vi "data_collector.vi"() -> ()   [LabVIEW 2024]
panel:
  out "Signal":dbl[](graph)
  in  "stop":bool
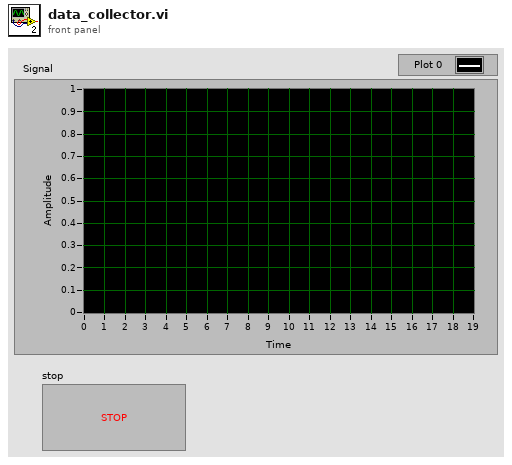
[diagram p1: front panel]
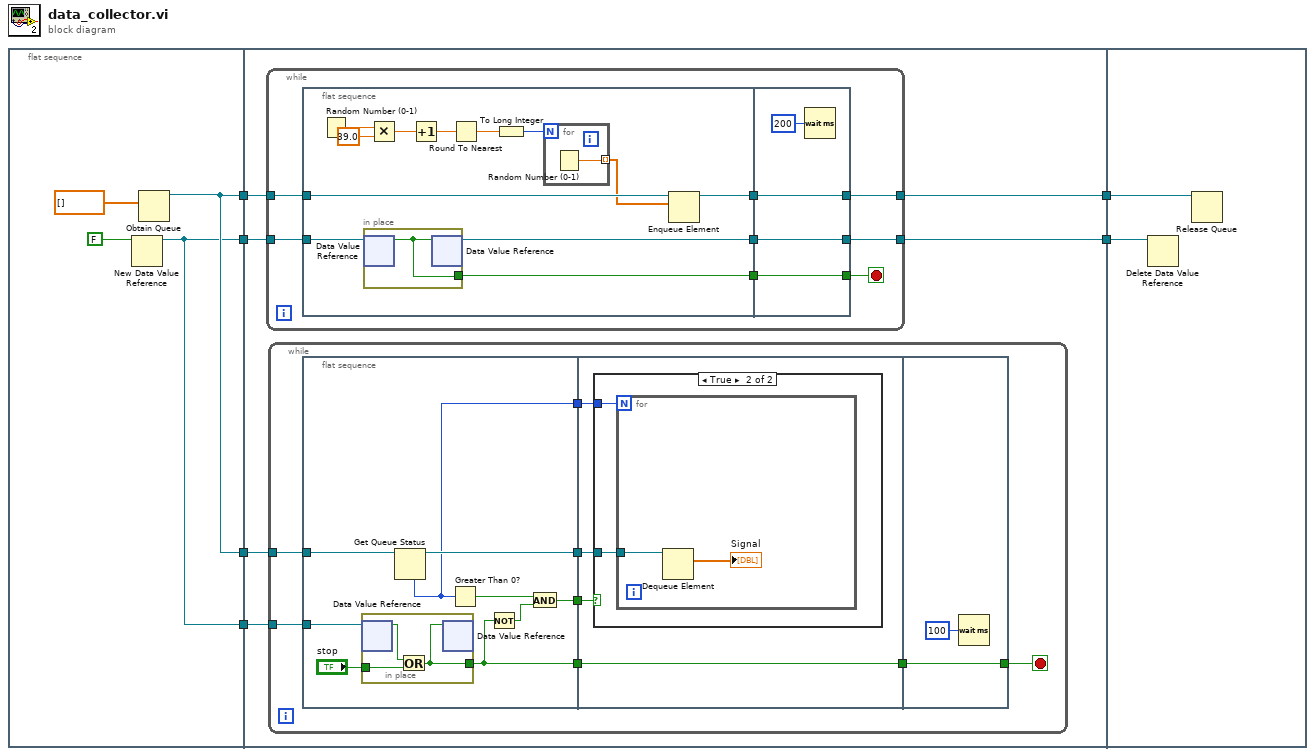
[diagram p0: block diagram]
diagram:
  n1 = flat-sequence {
    tunnel: [w8] -> w6
    tunnel: [w7] -> w5
    tunnel: [w8] -> w3
    tunnel: [w7] -> w2
    tunnel: w6 -> [w16]
    tunnel: w5 -> [w15]
    tunnel: [w14] -> w4
    tunnel: w3 -> [w13]
    tunnel: w2 -> [w12]
    tunnel: [w11] -> w1
    tunnel: w4 -> [w74]
    tunnel: w1 -> [w73]
    frame #0 {
      n2 = New Data Value Reference(data value=FALSE) -> (data value reference=w7:refnum<data-value>)  [unwired: 1 in, 1 out]
      n3 = Obtain Queue(element data type=dbl[] []) -> (queue out=w8:refnum<queue>)  [unwired: 4 in, 2 out]
    }
    frame #1 {
      n4 = while {
        tunnel: w16 -> [w53]
        tunnel: w15 -> [w54]
        tunnel: [w49] -> w14
        tunnel: [w47] -> w11
        stop <- w51 stop-if-true
        n5 = flat-sequence {
          tunnel: w54 -> [w58]
          tunnel: w53 -> [w60]
          tunnel: [w57] -> w52
          tunnel: [w56] -> w50
          tunnel: [w55] -> w48
          tunnel: [w71] -> w51
          tunnel: w52 -> [w71]
          tunnel: [w70] -> w49
          tunnel: w50 -> [w70]
          tunnel: w48 -> [w69]
          tunnel: [w69] -> w47
          frame #0 {
            n6 = Random Number (0-1)() -> (number: 0 to 1=w66:dbl)
            n7 = in-place {
              in-place-border: [w67] -> w57
              n8 = in-place-dvr #1(w58) -> (w67:bool)  [unwired: 1 out]
              n9 = in-place-dvr #1(w67) -> (w55:refnum<data-value>)  [unwired: 1 out]
            }
            n10 = Multiply(x=w66, y=39.0) -> (x*y=w64:dbl)
            n11 = Increment(x=w64) -> (x+1=w63:dbl)
            n12 = Round To Nearest(number=w63) -> (nearest integer value=w62:dbl)
            n13 = To Long Integer(number=w62) -> (32bit integer=w61:i32)
            n14 = for {
              N: w61 -> [_]
              tunnel: [w68] -> w59 mode=indexing
              n15 = Random Number (0-1)() -> (number: 0 to 1=w68:dbl)
            }
            n16 = Enqueue Element(queue=w60, element=w59) -> (queue out=w56:refnum<queue>)  [unwired: 2 in, 2 out]
          }
          frame #1 {
            n17 = Wait (ms)(milliseconds to wait=u32 200) -> ()  [unwired: 1 out]
          }
        }
      }
      n18 = while {
        tunnel: w13 -> [w24]
        tunnel: w12 -> [w23]
        stop <- w18 stop-if-true
        n19 = flat-sequence {
          tunnel: w24 -> [w31]
          tunnel: w23 -> [w33]
          tunnel: [w29] -> w22
          tunnel: [w26] -> w21
          tunnel: [w27] -> w20
          tunnel: [w25] -> w19
          tunnel: w22 -> [w37]
          tunnel: w21 -> [w40]
          tunnel: w20 -> [w39]
          tunnel: w19 -> [w38]
          tunnel: [w37] -> w17
          tunnel: [w46] -> w18
          tunnel: w17 -> [w46]
          frame #0 {
            n20 = in-place {
              in-place-border: "stop" -> [w36]
              in-place-border: [w34] -> w29
              n21 = in-place-dvr #2(w33) -> (w35:bool)  [unwired: 1 out]
              n22 = Or(x=w35, y=w36) -> (x .or. y?=w34:bool)
              n23 = in-place-dvr #2(w34) -> ()  [unwired: 2 out]
            }
            n24 = Get Queue Status(queue=w31) -> (queue out=w26:refnum<queue>, # elements in queue=w25:i32)  [unwired: 2 in, 6 out]
            n25 = Greater Than 0?(x=w25) -> (x > 0?=w30:bool)
            n26 = Not(x=w29) -> (.not. x?=w28:bool)
            n27 = And(x=w30, y=w28) -> (x .and. y?=w27:bool)
          }
          frame #1 {
            n28 = case shown="True" w39 {
              tunnel: w40 -> [_ w41]
              tunnel: w38 -> [_ w42]
              frame False {
              }
              frame True {
                n29 = for {
                  N: w42 -> [_]
                  tunnel: w41 -> [w44]
                  n30 = Dequeue Element(queue=w44) -> (element=→"Signal":dbl[])  [unwired: 2 in, 3 out]
                }
              }
            }
          }
          frame #2 {
            n31 = Wait (ms)(milliseconds to wait=u32 100) -> ()  [unwired: 1 out]
          }
        }
      }
    }
    frame #2 {
      n32 = Delete Data Value Reference(data value reference=w73) -> ()  [unwired: 1 in, 2 out]
      n33 = Release Queue(queue=w74) -> ()  [unwired: 2 in, 3 out]
    }
  }
